vi "savePharmaBotResults-v02.vi"(0 "controls array":refnum<vi>[](array[refnum]), 1 "protocol or memtest":enum16{"protocol", "memtest", "validation"}(ring), 2 "ExpPhase":string, 3 "which clamp":enum16{"VClamp", "IClamp"}(ring), 5 "protocol waveform":waveform(dbl)[](array[waveform]), 9 "protocol response":waveform(dbl)[](array[waveform]), 11 "error in":errorcluster caption="error in (no error)", 12 "metadata to save":T1 {"cell stats"."STD" format="%010.2f"; "cell stats"."Variance" format="%010.2f"; "cell stats"."Rt (MOhms)" format="%010.2f"; "cell stats"."tau (ms)" format="%08.2g"; "cell stats"."Cm (pF)" format="%08.2f"; "cell stats"."Ra (MOhms)" format="%010.2f"; "cell stats"."Rm (MOhms)" format="%010.2f"; "cell stats"."Ihold (pA)" format="%010.2f"}, 14 "Save to (folder dir)":path=path "C:/DATA/8-27-15 save func testing") -> (4 "controls array out":refnum<vi>[](array[refnum]), 15 "error out":errorcluster)   [LabVIEW 2019]
uses:
  autoWC/get_data_from_control_boolean.vi
  wc_protocol_v1.003 Folder/whole_cell_protocol/Controls/cell_stats-v02.ctl
  wc_protocol_v1.003 Folder/whole_cell_protocol/Controls/metadata_to_save.ctl
panel:
  out "rec path out":path
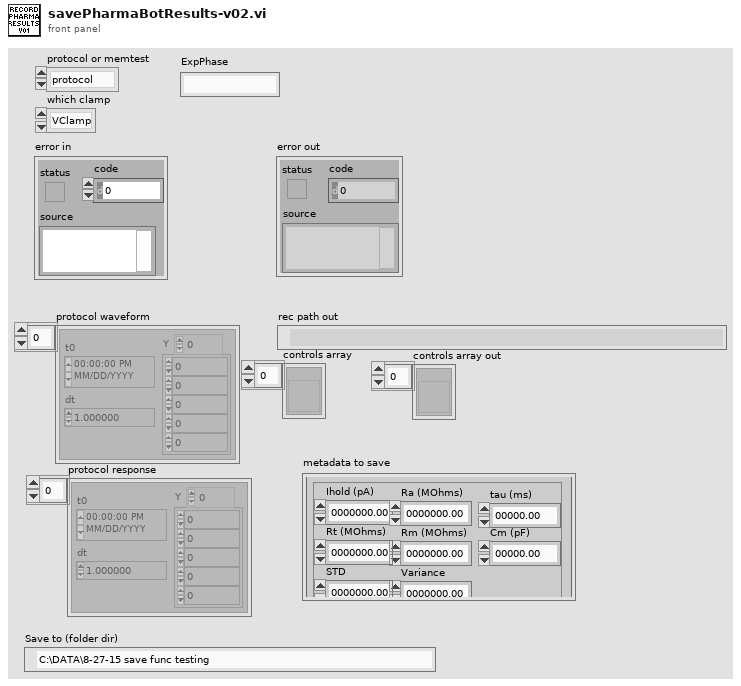
[diagram p1: front panel]
types:
  T1 = typedef "metadata_to_save.ctl" = cluster{"cell stats":T2}
  T2 = typedef "cell_stats-v02.ctl" = cluster{"Ihold (pA)":dbl, "Rm (MOhms)":dbl, "Ra (MOhms)":dbl, "Cm (pF)":dbl, "tau (ms)":dbl, "Rt (MOhms)":dbl, "Variance":dbl, "STD":dbl}
  T3 = enum16{"open", "replace", "create", "open or create", "replace or create", "replace or create with confirmation"}
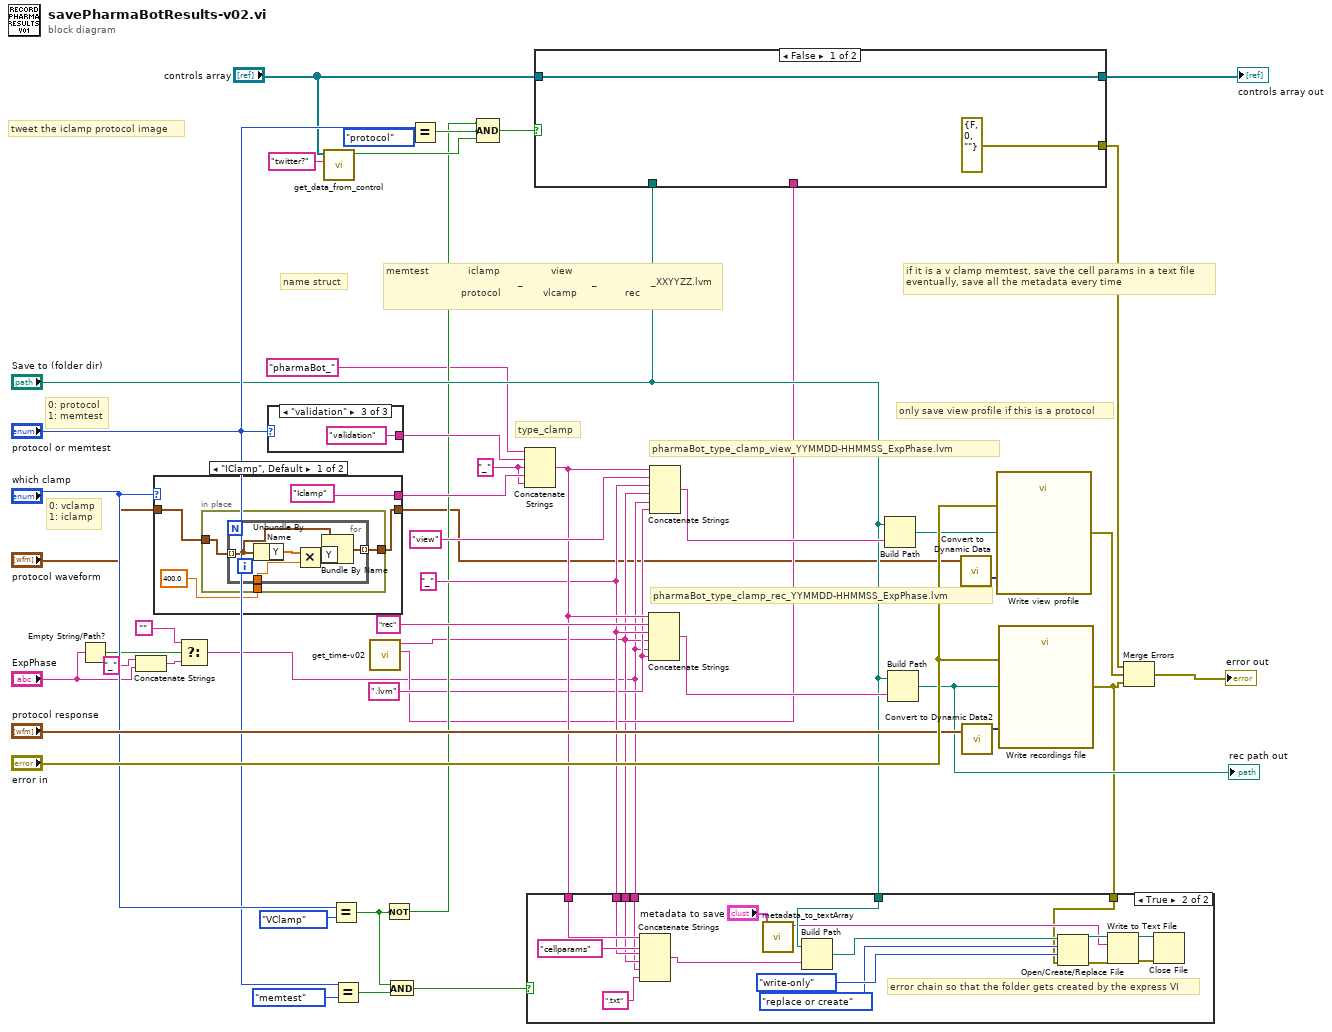
[diagram p0: block diagram]
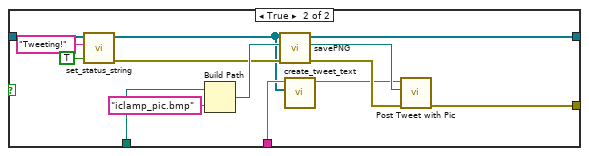
[diagram p2: hidden frame]
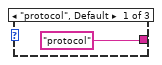
[diagram p4: hidden frame]
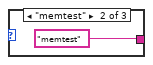
[diagram p5: hidden frame]
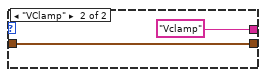
[diagram p6: hidden frame]
diagram:
  w12 = ".lvm" ("name or relative path")
  w27 = "_" ("string")
  w41 = "_" ("string")
  # "tweet the iclamp protocol image"
  # "if it is a v clamp memtest, save the cell params in a text file\neventually, save all the metadata every time"
  # "only save view profile if this is a protocol"
  # "pharmaBot_type_clamp_rec_YYMMDD-HHMMSS_ExpPhase.lvm"
  # "pharmaBot_type_clamp_view_YYMMDD-HHMMSS_ExpPhase.lvm"
  # "type_clamp"
  # "name struct"
  # "memtest             iclamp                 view            \n                                            _                       _                  _XXYYZZ.lvm\n                         protocol              vlcamp                rec"
  # "0: protocol\n1: memtest"
  # "0: vclamp\n1: iclamp"
  n1 = Empty String/Path?(string/path="ExpPhase") -> (empty?=w11:bool)
  n2 = Concatenate Strings("_" ("string"), "ExpPhase") -> (w8:string)
  n3 = case shown="\"IClamp\", Default" "which clamp" {
    tunnel: ["Iclamp" "Vclamp"] -> w42
    tunnel: "protocol waveform" -> [w50 w60]
    tunnel: [w49 w60] -> w1
    frame "IClamp", Default {
      n4 = in-place {
        in-place-border: w50 -> [w54]
        in-place-border: [w53] -> w49
        in-place-border: 400.0 -> [w52]
        n5 = for {
          tunnel: w54 -> [w59] mode=indexing
          tunnel: [w58] -> w53 mode=indexing
          tunnel: w52 -> [w55]
          n6 = Unbundle By Name(w59) -> ("Y"=w57:dbl[])
          n7 = Multiply(x=w57, y=w55) -> (x*y=w56:dbl[])
          n8 = Bundle By Name(cluster=w59, "Y"=w56) -> (w58:waveform(dbl))
        }
      }
    }
    frame "VClamp" {
    }
  }
  n9 = Select(t="", s=w11, f=w8) -> (s? t:f=w3:string)
  n10 = case shown="\"validation\"" "protocol or memtest" {
    tunnel: ["protocol" "memtest" "validation"] -> w43
    frame "protocol", Default {
    }
    frame "memtest" {
    }
    frame "validation" {
    }
  }
  n11 = call-poly "get_data_from_control.vi"("control label"="twitter?", "controls array"="controls array") -> ("Boolean"=w18:bool)  [unwired: 8 in, 1 out]
  n12 = Equal?(x="which clamp", y=enum16{"VClamp", "IClamp"}."VClamp") -> (x = y?=w14:bool)
  n13 = Equal?(x="protocol or memtest", y=enum16{"protocol", "memtest"}."memtest") -> (x = y?=w16:bool)
  n14 = call "get_time-v02.vi"() -> ("time output"=w5:string, "pure text output"=w4:string)  [unwired: 10 in]
  n15 = Not(x=w14) -> (.not. x?=w13:bool)
  n16 = And(x=w14, y=w16) -> (x .and. y?=w29:bool)
  n17 = Equal?(x="protocol or memtest", y=enum16{"protocol", "memtest"}."protocol") -> (x = y?=w23:bool)
  n18 = Compound Arithmetic op=AND(w13, w23, w18) -> (w22:bool)
  n19 = Concatenate Strings("pharmaBot_" ("string"), w43, w41, w42, w41) -> (w28:string)
  n20 = case shown="False" w22 {
    tunnel: "controls array" -> [w66 w71]
    tunnel: [w66 w76] -> w21
    tunnel: "Save to (folder dir)" -> [_ w80]
    tunnel: [errorcluster {"status"=FALSE, "code"=0, "source"=""} ("error out") w74] -> w15
    tunnel: w5 -> [_ w73]
    frame False {
    }
    frame True {
      n21 = call "set_status_string.vi"("new line?"=TRUE, "status string in"="Tweeting!", "controls array"=w71) -> ("error out"=w70:errorcluster, "controls array out"=w67:refnum<vi>[])  [unwired: 7 in]
      n22 = Build Path(base path=w80, name or relative path="iclamp_pic.bmp") -> (appended path=w79:path)
      n23 = call "savePNG.vi"("error in"=w70, "image path in (.bmp)"=w79, "controls array in"=w67) -> ("error out"=w75:errorcluster, "image path out (.PNG)"=w77:path, "controls array out"=w76:refnum<vi>[])  [unwired: 6 in]
      n24 = call "create_tweet_text.vi"("controls array"=w67, "time string"=w73) -> ("tweet"=w72:string)  [unwired: 9 in]
      n25 = call "Post Tweet with Pic.vi"("error in"=w75, "Picture File (PNG, JPG, GIF)"=w77, "Tweet"=w72) -> ("error out"=w74:errorcluster)  [unwired: 8 in]
    }
  }
  "controls array out" <- w21
  n26 = Concatenate Strings(w28, "rec" ("name or relative path"), w27, w4, w3, w12) -> (w37:string)
  n27 = Concatenate Strings(w28, "view" ("name or relative path"), w27, w4, w3, w12) -> (w38:string)
  n28 = Build Path(base path="Save to (folder dir)", name or relative path=w38) -> (appended path=w33:path)
  n29 = Build Path(base path="Save to (folder dir)", name or relative path=w37) -> (appended path=w35:path)
  "rec path out" <- w35
  n30 = call "Convert to Dynamic Data"("Array of Waveforms"=w1) -> ("Dynamic Data Type"=w34:dynamicdata)  [unwired: 3 in]
  n31 = call "Convert to Dynamic Data2"("Array of Waveforms"="protocol response") -> ("Dynamic Data Type"=w47:dynamicdata)  [unwired: 3 in]
  n32 = call "Write view profile"("Signals"=w34, "error in (no error)"="error in", "Filename"=w33) -> ("error out"=w45:errorcluster)  [unwired: 14 in, 2 out]
  n33 = call "Write recordings file"("Signals"=w47, "error in (no error)"="error in", "Filename"=w35) -> ("error out"=w26:errorcluster)  [unwired: 14 in, 2 out]
  n34 = case shown="True" w29 {
    tunnel: "Save to (folder dir)" -> [_ w93]
    tunnel: w28 -> [_ w91]
    tunnel: w27 -> [_ w89]
    tunnel: w4 -> [_ w88]
    tunnel: w26 -> [_ w83]
    tunnel: w3 -> [_ w82]
    frame False {
    }
    frame True {
      # "error chain so that the folder gets created by the express VI"
      n35 = Concatenate Strings(w91, "cellparams" ("name or relative path"), w89, w88, w82, ".txt" ("name or relative path")) -> (w92:string)
      n36 = call "metadata_to_textArray.vi"("metadata to save"="metadata to save") -> ("xml string out"=w86:string)  [unwired: 10 in]
      n37 = Build Path(base path=w93, name or relative path=w92) -> (appended path=w94:path)
      n38 = Open/Create/Replace File(file path (use dialog)=w94, error in=w83, operation (0:open)=T3."replace or create", access (0:read/write)=enum16{"read/write", "read-only", "write-only"}."write-only") -> (refnum out=w95:refnum<file>, error out=w97:errorcluster)  [unwired: 2 in, 1 out]
      n39 = Write to Text File(file (use dialog)=w95, text=w86, error in=w97) -> (refnum out=w85:refnum<file>, error out=w96:errorcluster)  [unwired: 1 in, 1 out]
      n40 = Close File(refnum=w85, error in=w96) -> ()  [unwired: 2 out]
    }
  }
  n41 = Merge Errors(w15, w45, w26) -> (→"error out":errorcluster)
